vi "regular expression to csv.vi"(11 "regular expression":string) -> (3 "csv":string)   [LabVIEW 2013, in "control module data interface generator.lvlib"]
uses:
  <vilib>/regexp/Match Regular Expression.xnode
  control module data interface generator.lvlib
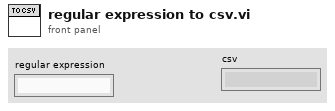
[diagram p1: front panel]
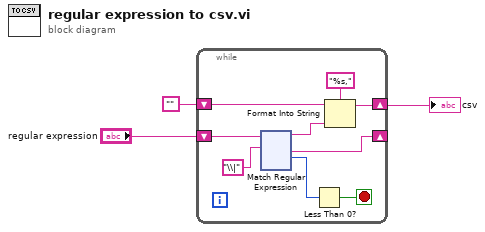
[diagram p0: block diagram]
diagram:
  n1 = while {
    shift-right: [w9] -> _
    shift-left: "regular expression" -> [w12]
    shift-right: [w4] -> w1
    shift-left: "" -> [w7]
    stop <- w8 stop-if-true
    n2 = xnode "Match Regular Expression"("input string"=w12, "regular expression"="\\|") -> ("before match"=w5:string, "after match"=w9:string, "offset past match"=w10:i32)  [unwired: 4 in, 2 out]
    n3 = Less Than 0?(x=w10) -> (x < 0?=w8:bool)
    n4 = Format Into String(format string="%s,", initial string=w7, w5) -> (resulting string=w4:string)  [unwired: 1 in, 1 out]
  }
  "csv" <- w1
